vi "CloseXL_Worksheet.vi"(8 "error in (no error)":errorcluster, 11 "Refnum Cluster In":T1) -> (0 "error out":errorcluster, 3 "Refnum Cluster Out":T2)   [LabVIEW 2017, in "excel_configuration.lvlib"]
doc: "Closes the open Excel worksheet and releases its ActiveX reference."
uses:
  excel_configuration.lvlib
  492f34d0-45a3-4e32-b986-c7fb35302db1.vi
  ed38021d-5bf3-40fc-9641-79566d57dbf5.vi
  <vilib>/Utility/error.llb/Clear Errors.vi
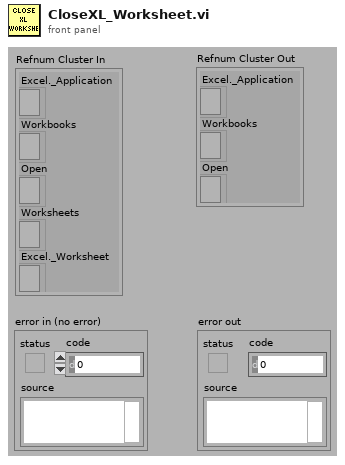
[diagram p1: front panel]
types:
  T1 = cluster{"Excel._Application":refnum<k7>, "Workbooks":refnum<k7>, "Open":refnum<k7>, "Worksheets":refnum<k7>, "Excel._Worksheet":refnum<k7>}
  T2 = cluster{"Excel._Application":refnum<k7>, "Workbooks":refnum<k7>, "Open":refnum<k7>}
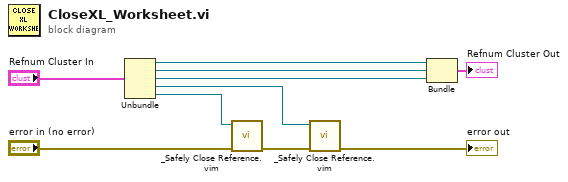
[diagram p0: block diagram]
diagram:
  n1 = Unbundle("Refnum Cluster In") -> ("Excel._Application"=w7:refnum<k7>, "Workbooks"=w8:refnum<k7>, "Open"=w9:refnum<k7>, "Worksheets"=w3:refnum<k7>, "Excel._Worksheet"=w4:refnum<k7>)
  n2 = call "_Safely Close Reference.vim"("error in (no error)"="error in (no error)", "Automation Refnum in"=w4) -> ("error out"=w2:errorcluster)  [unwired: 9 in]
  n3 = call "_Safely Close Reference.vim"("error in (no error)"=w2, "Automation Refnum in"=w3) -> ("error out"=→"error out":errorcluster)  [unwired: 9 in]
  n4 = Bundle("Excel._Application"=w7, "Workbooks"=w8, "Open"=w9) -> (→"Refnum Cluster Out":T2)  [unwired: 1 in]
